vi "Read Matlab Params.vi"(8 "error in (no error)":errorcluster, 10 "Enum":T1(ring), 11 "TrialBasedExperiment in":refnum<class "WNOriDiscExperiment.lvclass">) -> (0 "error out":errorcluster, 2 "Matlab Param Array":cluster{"Name":string, "Data":variant}[](array[cluster]), 3 "TrialBasedExperiment out":refnum<class "WNOriDiscExperiment.lvclass">)   [LabVIEW 2011, in "WNOriDiscExperiment.lvclass"]
uses:
  WNOriDiscExperiment.lvclass
  TwoAfcEye/TwoAfcEye.lvclass
  WNOriDiscExperiment.lvclass/WNOriDiscExperiment.ctl
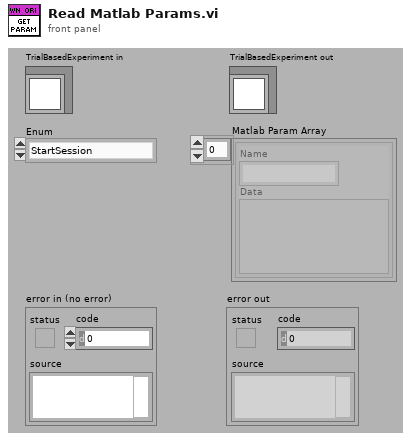
[diagram p1: front panel]
types:
  T1 = enum16{"StartSession", "StartTrial", "ShowStimulus"}
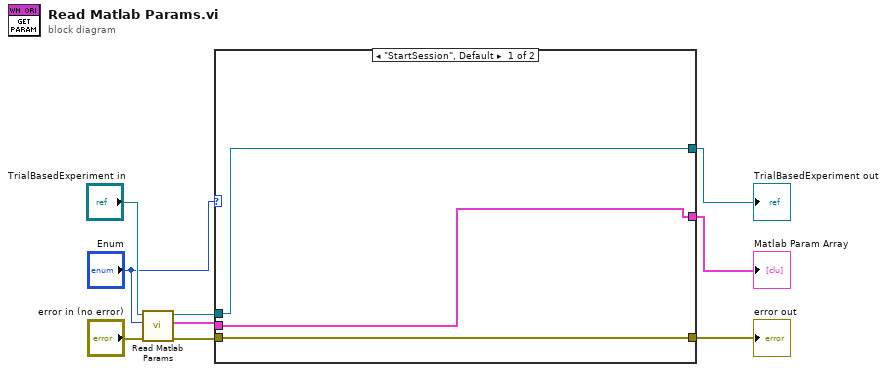
[diagram p0: block diagram]
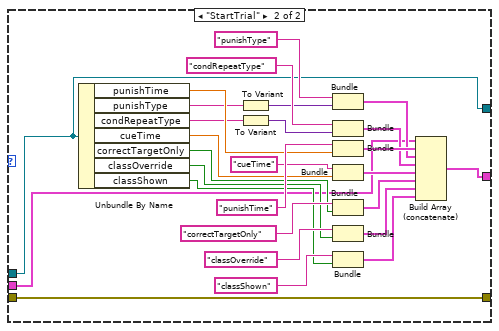
[diagram p2: hidden frame]
diagram:
  n1 = call-parent "Read Matlab Params.vi"("error in (no error)"="error in (no error)", "Enum"="Enum", "TrialBasedExperiment in"="TrialBasedExperiment in") -> ("error out"=w5:errorcluster, "Matlab Param Array"=w6:cluster{"Name":string, "Data":variant}[], "TrialBasedExperiment out"=w7:refnum<class "WNOriDiscExperiment.lvclass">)  [unwired: 6 in]
  n2 = case shown="\"StartSession\", Default" "Enum" {
    tunnel: w7 -> [w12 w14]
    tunnel: w5 -> [w11 w15]
    tunnel: [w10 w16] -> w2
    tunnel: [w11 w15] -> w1
    tunnel: [w12 w14] -> w3
    tunnel: w6 -> [w10 w13]
    frame "StartSession", Default {
    }
    frame "StartTrial" {
      n3 = Unbundle By Name(w14) -> ("punishTime"=w35:dbl, "punishType"=w32:string, "condRepeatType"=w30:string, "cueTime"=w27:dbl, "correctTargetOnly"=w24:bool, "classOverride"=w20:bool, "classShown"=w19:bool)
      n4 = To Variant(anything=w32) -> (Variant=w33:variant)
      n5 = To Variant(anything=w30) -> (Variant=w31:variant)
      n6 = Bundle("punishType", "Variant"=w33) -> (w34:cluster{string, "Variant":variant})  [unwired: 1 out]
      n7 = Bundle("condRepeatType", "Variant"=w31) -> (w29:cluster{string, "Variant":variant})  [unwired: 1 out]
      n8 = Bundle("punishTime", "punishTime"=w35) -> (w37:cluster{string, "punishTime":dbl})  [unwired: 1 out]
      n9 = Bundle("cueTime", "cueTime"=w27) -> (w26:cluster{string, "cueTime":dbl})  [unwired: 1 out]
      n10 = Bundle("correctTargetOnly", "correctTargetOnly"=w24) -> (w23:cluster{string, "correctTargetOnly":bool})  [unwired: 1 out]
      n11 = Bundle("classOverride", "classOverride"=w20) -> (w18:cluster{string, "classOverride":bool})  [unwired: 1 out]
      n12 = Bundle("classShown", "classShown"=w19) -> (w17:cluster{string, "classShown":bool})  [unwired: 1 out]
      n13 = Build Array (concatenate)(w13, w37, w34, w29, w26, w23, w18, w17) -> (w16:cluster{"Name":string, "Variant":variant}[])
    }
  }
  "error out" <- w1
  "TrialBasedExperiment out" <- w3
  "Matlab Param Array" <- w2
